vi "citTemplate.ErrorEventPass.vi"(5 "ignore error (F)":bool, 7 "instance":i32, 8 "error in":errorcluster, 10 "action of error":variant, 11 "event in":variant) -> (0 "error out":errorcluster)   [LabVIEW 2016]
uses:
  citTemplate.errData.ctl
  EventLog/EventLog.EventSource.ctl
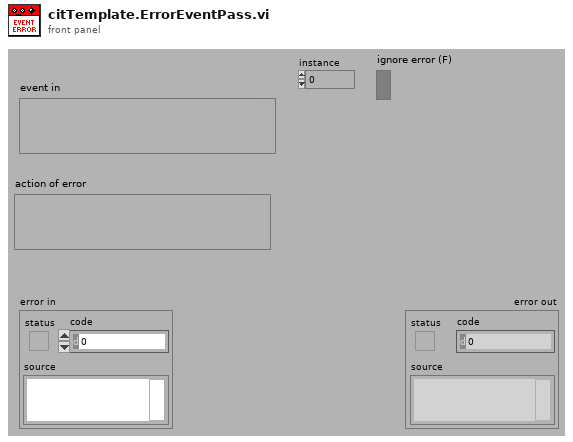
[diagram p1: front panel]
types:
  T1 = typedef "citTemplate.errData.ctl" = cluster{"ts":timestamp, "src":T2, "instance":i32, "action":string, "error":errorcluster, "unconfirmed":bool}
  T2 = typedef "EventLog.EventSource.ctl" = enum16{"All", "Gui", "Cache", "PLC1", "PLC2", "PLC3", "DB", "DB01", "DB02", "DB03", "DB04", "DB05", "DB06", "DB07", "DB08", "DB09", "DB10", "DB11", "DB12", "DB13", "DB14", "DB15", "DB16"}
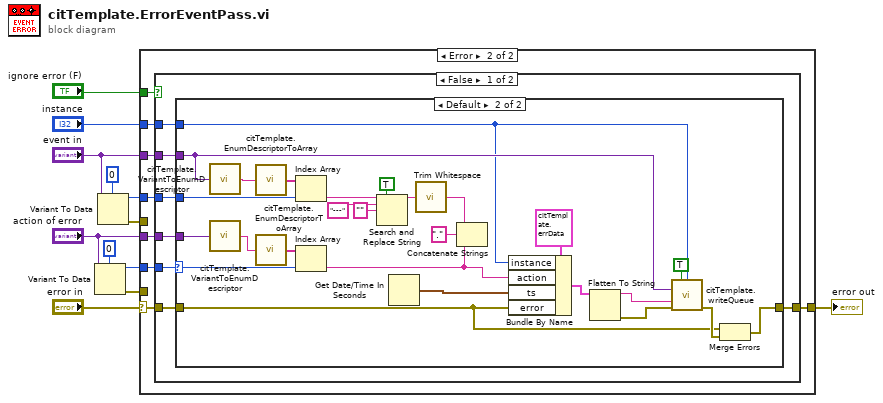
[diagram p0: block diagram]
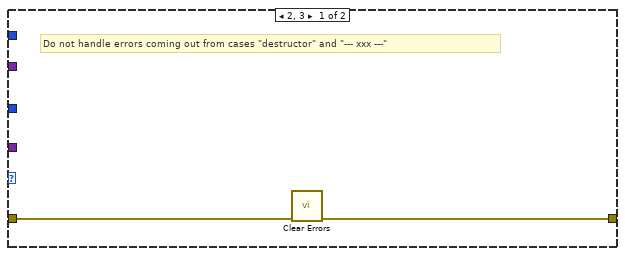
[diagram p3: hidden frame]
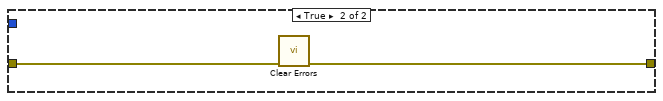
[diagram p4: hidden frame]
diagram:
  n1 = Variant To Data(type=u32 0 ("u32"), Variant="action of error") -> (data=w8:u32, error out=w9:errorcluster)  [unwired: 1 in]
  n2 = Variant To Data(type=u32 0 ("u32"), Variant="event in") -> (data=w5:u32, error out=w6:errorcluster)  [unwired: 1 in]
  n3 = case shown="Error" "error in" {
    selector: "error in" -> [w13 w17]
    tunnel: [w13 w21] -> w11
    tunnel: "event in" -> [_ w20]
    tunnel: "action of error" -> [_ w19]
    tunnel: w9 -> [_ _]
    tunnel: w8 -> [_ w15]
    tunnel: w6 -> [_ _]
    tunnel: w5 -> [_ w18]
    tunnel: "instance" -> [_ w16]
    tunnel: "ignore error (F)" -> [_ w14]
    frame No Error {
    }
    frame Error {
      n4 = case shown="False" w14 {
        tunnel: [w28 w57] -> w21
        tunnel: w20 -> [w27 _]
        tunnel: w19 -> [w26 _]
        tunnel: w18 -> [w25 _]
        tunnel: w17 -> [w24 w58]
        tunnel: w16 -> [w23 _]
        tunnel: w15 -> [w22 _]
        frame False {
          n5 = case shown="Default" w22 {
            selector: w22 -> [_ w44]
            tunnel: [w29 w34] -> w28
            tunnel: w27 -> [_ w51]
            tunnel: w26 -> [_ w50]
            tunnel: w25 -> [_ w45]
            tunnel: w24 -> [w30 w33]
            tunnel: w23 -> [_ w35]
            frame 2, 3 {
              # "Do not handle errors coming out from cases \"destructor\" and \"--- xxx ---\""
              n6 = call <vilib>:"Clear Errors.vi"("error in (no error)"=w30) -> ("error out"=w29:errorcluster)  [unwired: 5 in, 1 out]
            }
            frame Default {
              n7 = call "citTemplate.VariantToEnumDescriptor.vi"("Variant enum data"=w51) -> ("enum type descriptor"=w46:string)  [unwired: 14 out]
              n8 = call "citTemplate.VariantToEnumDescriptor.vi"("Variant enum data"=w50) -> ("enum type descriptor"=w49:string)  [unwired: 14 out]
              n9 = call "citTemplate.EnumDescriptorToArray.vi"("enum type descriptor"=w46) -> ("array"=w47:string[])  [unwired: 14 out]
              n10 = call "citTemplate.EnumDescriptorToArray.vi"("enum type descriptor"=w49) -> ("array"=w48:string[])  [unwired: 14 out]
              n11 = Index Array(array=w47, index=w45) -> (element=w42:string)
              n12 = Index Array(array=w48, index=w44) -> (element=w32:string)
              n13 = Search and Replace String(replace all?=TRUE ("replace all? (F)"), input string=w42, search string="---" ("substring (\"\")"), replace string="" ("replace string (\"\")")) -> (result string=w41:string)  [unwired: 4 in, 3 out]
              n14 = Get Date/Time In Seconds() -> (seconds since 1Jan1904=w31:timestamp)
              n15 = call <vilib>:"Trim Whitespace.vi"("string"=w41) -> ("trimmed string"=w37:string)  [unwired: 1 in]
              n16 = Concatenate Strings(w37, "." ("string"), w32) -> ()  [unwired: 1 out]
              n17 = Bundle By Name(cluster=T1 {"ts"=timestamp(0 s since 1904-01-01), "src"=enum."All", "instance"=0, "action"="", "error"={"status"=FALSE, "code"=0, "source"=""}, "unconfirmed"=FALSE} ("ErrData"), "instance"=w35, "action"=w32, "ts"=w31, "error"=w33) -> (w53:T1)
              n18 = Flatten To String(anything=w53) -> (data string=w54:string, error out=w55:errorcluster)  [unwired: 2 in, 2 out]
              n19 = call "citTemplate.writeQueue.vi"("High priority (F)"=TRUE, "instance (0)"=w35, "event in (if not connected:all statemachine with data event)"=w51, "data in"=w54, "error in (no error)"=w55) -> ("error out"=w56:errorcluster)  [unwired: 10 out]
              n20 = Merge Errors(w33, w56) -> (w34:errorcluster)
            }
          }
        }
        frame True {
          n21 = call <vilib>:"Clear Errors.vi"("error in (no error)"=w58) -> ("error out"=w57:errorcluster)  [unwired: 5 in, 1 out]
        }
      }
    }
  }
  "error out" <- w11
